vi "Create (New).vi"(6 "Config Version (0.0.0)":string="0.0.0", 8 "error in (no error)":errorcluster) -> (0 "error out":errorcluster, 3 "VolatusConfig out":refnum<class "VolatusConfig.lvclass">)   [LabVIEW 2023, in "VolatusConfig.lvlib" / "VolatusConfig.lvclass"]
uses:
  VolatusConfig.lvclass
  VolatusConfig.lvclass/VolatusConfig.ctl
  lv-cdm/CDM-Config/Config Manager/Config Manager.lvclass
  lv-cdm/CDM-Config/Config Element/Config Element.lvclass
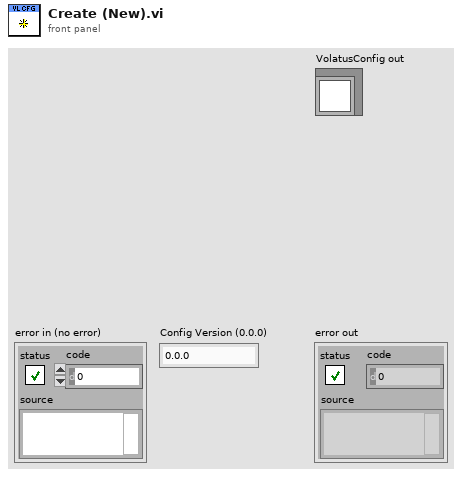
[diagram p1: front panel]
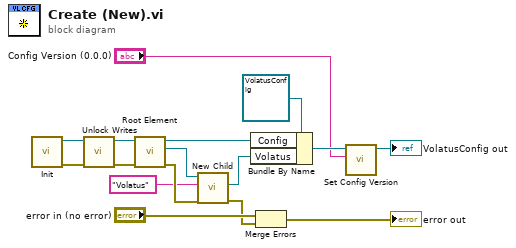
[diagram p0: block diagram]
diagram:
  n1 = call "Init.vi"() -> ("error out"=w10:errorcluster, "Config Manager out"=w2:refnum<class "Config Manager.lvclass">)  [unwired: 10 in]
  n2 = call "Unlock Writes.vi"("error in (no error)"=w10, "Config Manager in"=w2) -> ("error out"=w3:errorcluster, "Config Manager out"=w1:refnum<class "Config Manager.lvclass">)  [unwired: 8 in]
  n3 = call "Root Element.vi"("error in (no error)"=w3, "Config Manager in"=w1) -> ("error out"=w16:errorcluster, "Root Element"=w12:refnum<class "Config Element.lvclass">, "Config Manager out"=w13:refnum<class "Config Manager.lvclass">)  [unwired: 7 in]
  n4 = call "New Child.vi"("error in (no error)"=w16, "Child Name"="Volatus", "Config Element in"=w12) -> ("error out"=w5:errorcluster, "New Child"=w4:refnum<class "Config Element.lvclass">)  [unwired: 6 in, 1 out]
  n5 = Bundle By Name(cluster=refnum<class "VolatusConfig.lvclass"> refnum ("VolatusConfig in"), "Config"=w13, "Volatus"=w4) -> (w8:refnum<class "VolatusConfig.lvclass">)
  n6 = Merge Errors("error in (no error)", w5) -> (→"error out":errorcluster)
  n7 = call "Set Config Version.vi"("Config Version"="Config Version (0.0.0)", "VolatusConfig in"=w8) -> ("VolatusConfig out"=→"VolatusConfig out":refnum<class "VolatusConfig.lvclass">)  [unwired: 8 in, 1 out]
